vi "Get Variant.vi"(7 "PV name":string, 8 "error in":errorcluster, 9 "timeout":dbl[unit]=1.0, 11 "Client in":refnum<class "Client.lvclass">) -> (0 "error out":errorcluster, 1 "timed out?":bool, 2 "value":variant, 3 "Client out":refnum<class "Client.lvclass">, 5 "timestamp":timestamp)   [LabVIEW 2020, in "Client.lvlib" / "Client.lvclass"]
doc: "Get a value from a PV.\n\nThe input <B>default</B> must either\n- A value matching the type of the PV, the output <B>value</B> will be the same type\n- A type code matching the type of the PV, <B>value</B> will be a variant\n- A variant containing a value matching the type of the PV, <B>value</B> will be a variant"
uses:
  Client.lvclass
  Client.lvclass/Client.ctl
  Value/Value/Value.lvclass
  64639a28-9dc2-4f97-896e-9c20cd4f45be.vi
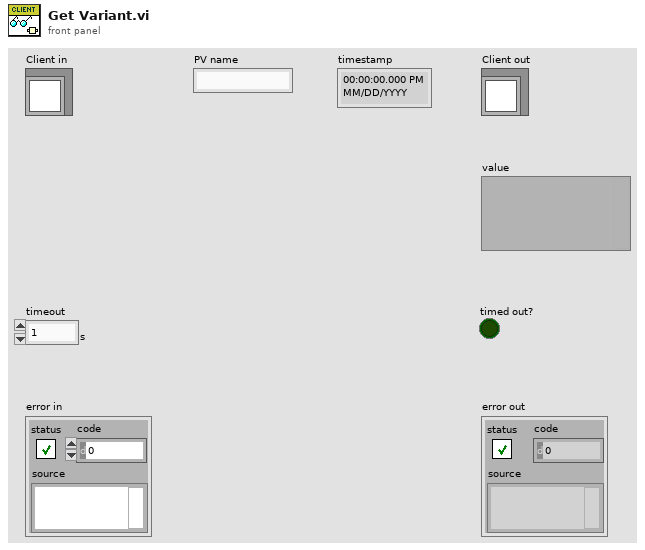
[diagram p1: front panel]
types:
  T1 = typedef "Value.lvlib/Display Metadata.ctl" = cluster{"Limit Low":dbl, "Limit High":dbl, "Description":string, "Units":string, "Precision":i32, "Form":enum32{"Default", "String", "Binary", "Decimal", "Hex", "Exponential", "Engineering"}}
  T2 = typedef "Value.lvlib/Alarm Status.ctl" = cluster{"Severity":enum32{"no", "minor", "major", "record", "invalid", "undefined", ""}, "Status":enum32{"no", "device", "driver", "record", "db", "conf", "undefined", "client"}, "Message":string}
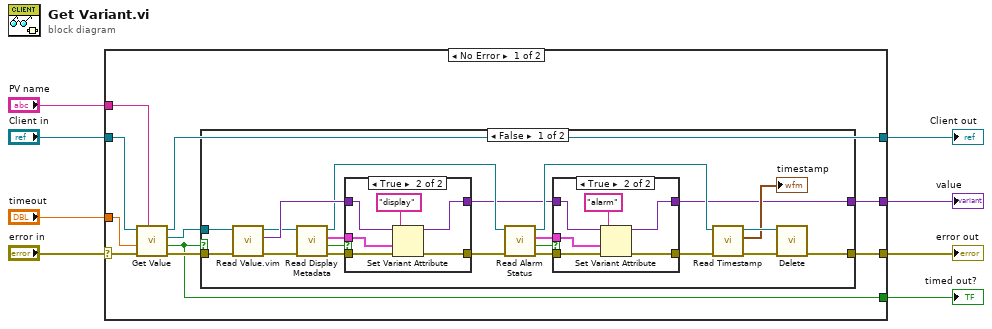
[diagram p0: block diagram]
diagram:
  n1 = case shown="No Error" "error in" {
    selector: "error in" -> [w16 w57]
    tunnel: [w13 w57] -> w3
    tunnel: [w12 w58] -> w4
    tunnel: "Client in" -> [w18 w58]
    tunnel: "PV name" -> [w17 _]
    tunnel: "timeout" -> [w9 _]
    tunnel: [w11 _] -> w2
    tunnel: [w10 _] -> w1
    frame No Error {
      n2 = call "Get Value.vi"("PV name"=w17, "error in"=w16, "timeout"=w9, "Client in"=w18) -> ("error out"=w15:errorcluster, "timed out?"=w11:bool, "Value out"=w14:refnum<class "Value.lvclass">, "Client out"=w12:refnum<class "Client.lvclass">)  [unwired: 4 in]
      n3 = case shown="False" w11 {
        tunnel: w15 -> [w38 w56]
        tunnel: w14 -> [w37 _]
        tunnel: [w39 w56] -> w13
        tunnel: [w19 _] -> w10
        frame False {
          n4 = call "Read Value.vim"("error in"=w38, "Value in"=w37) -> ("error out"=w36:errorcluster, "value"=w32:variant, "Value out"=w31:refnum<class "Value.lvclass">)  [unwired: 6 in, 1 out]
          n5 = call "Read Display Metadata.vi"("error in"=w36, "Value in"=w31) -> ("error out"=w34:errorcluster, "has display metadata?"=w35:bool, "display metadata"=w33:T1, "Value out"=w25:refnum<class "Value.lvclass">)  [unwired: 6 in]
          n6 = case shown="True" w35 {
            tunnel: w34 -> [w49 w55]
            tunnel: [w49 w54] -> w27
            tunnel: w33 -> [_ w53]
            tunnel: w32 -> [w48 w52]
            tunnel: [w48 w50] -> w21
            frame False {
            }
            frame True {
              n7 = Set Variant Attribute(Variant=w52, name="display", value=w53, error in=w55) -> (Variant out=w50:variant, error out=w54:errorcluster)  [unwired: 1 out]
            }
          }
          n8 = call "Read Alarm Status.vi"("error in"=w27, "Value in"=w25) -> ("error out"=w26:errorcluster, "has alarm status?"=w22:bool, "alarm status"=w23:T2, "Value out"=w24:refnum<class "Value.lvclass">)  [unwired: 6 in]
          n9 = case shown="True" w22 {
            tunnel: w26 -> [w41 w47]
            tunnel: [w41 w46] -> w20
            tunnel: w23 -> [_ w45]
            tunnel: w21 -> [w40 w42]
            tunnel: [w40 w43] -> w19
            frame False {
            }
            frame True {
              n10 = Set Variant Attribute(Variant=w42, name="alarm", value=w45, error in=w47) -> (Variant out=w43:variant, error out=w46:errorcluster)  [unwired: 1 out]
            }
          }
          n11 = call "Read Timestamp.vi"("error in"=w20, "Value in"=w24) -> ("error out"=w30:errorcluster, "timestamp"=→"timestamp":timestamp, "Value out"=w29:refnum<class "Value.lvclass">)  [unwired: 7 in]
          n12 = call "Delete.vi"("error in (no error)"=w30, "Value in"=w29) -> ("error out"=w39:errorcluster)  [unwired: 9 in]
        }
        frame True {
        }
      }
    }
    frame Error {
    }
  }
  "error out" <- w3
  "Client out" <- w4
  "value" <- w1
  "timed out?" <- w2
